vi "Read LUT Ref.vi"(8 "error in (no error)":errorcluster, 11 "LUT in":refnum<class "LUT.lvclass">) -> (0 "error out":errorcluster, 2 "LUT Ref":refnum<data-value>, 3 "LUT out":refnum<class "LUT.lvclass">)   [LabVIEW 2017, in "LUT.lvlib" / "LUT.lvclass"]
doc: "Returns the look up tabel (LUT) reference."
uses:
  LUT.lvclass
  LUT.lvclass/LUT.ctl
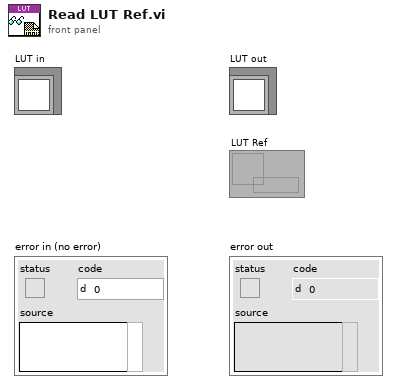
[diagram p1: front panel]
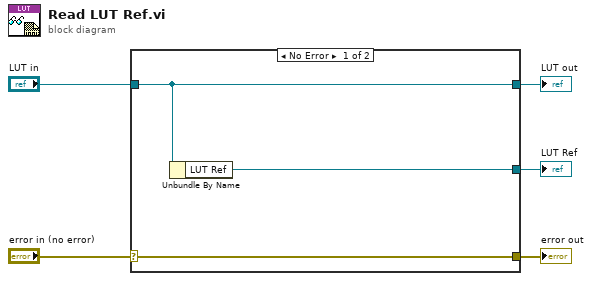
[diagram p0: block diagram]
diagram:
  n1 = case shown="No Error" "error in (no error)" {
    selector: "error in (no error)" -> [w8 w9]
    tunnel: [w8 w9] -> w4
    tunnel: [w7 w10] -> w2
    tunnel: "LUT in" -> [w7 w10]
    tunnel: [w6 _] -> w1
    frame No Error {
      n2 = Unbundle By Name(w7) -> ("LUT Ref"=w6:refnum<data-value>)
    }
    frame Error {
    }
  }
  "error out" <- w4
  "LUT out" <- w2
  "LUT Ref" <- w1
